vi "GenCtrlCsv.vi"(6 "Loop Time (s)":dbl, 7 "Gen Control":T1, 8 "error in (no error)":errorcluster, 9 "ROSCO Params in":T6, 10 "IO Signals In":T5, 11 "ArrayPairs In":T3={"iStatus"={"Index"=0, "Value"=0.0}, "TIME"={"Index"=1, "Value"=0.0}, "DT"={"Index"=2, "Value"=0.0}, "Blade1PitchPos_rad"={"Index"=3, "Value"=0.0}, "VS_MECHGENPWR"={"Index"=13, "Value"=0.0}, "VS_GENPWR"={"Index"=14, "Value"=0.0}, "GEN_SPEED"={"Index"=19, "Value"=0.0}, "ROTOR_SPEED"={"Index"=20, "Value"=0.0}, "GENTQMEAS"={"Index"=22, "Value"=0.0}, "Y_M"={"Index"=23, "Value"=0.0}, "HORWINDV"={"Index"=26, "Value"=0.0}, "ROOTMOOP1"={"Index"=29, "Value"=0.0}, "ROOTMOOP2"={"Index"=30, "Value"=0.0}, "Blade2PitchPos_rad"={"Index"=32, "Value"=0.0}, "Blade3PitchPos_rad"={"Index"=33, "Value"=0.0}, "ROOTMOOP3"={"Index"=31, "Value"=0.0}, "AVCMSG_SIZE"={"Index"=48, "Value"=0.0}, "INFILE_SIZE "={"Index"=49, "Value"=0.0}, "OUTFILE_SIZE "={"Index"=50, "Value"=0.0}, "FA_ACC"={"Index"=52, "Value"=0.0}, "NUM_BLADES"={"Index"=60, "Value"=0.0}, "BladePitchSetpoint_rad"={"Index"=44, "Value"=0.0}, "TorqueSetpoint_Nm"={"Index"=46, "Value"=0.0}, "OUT_AEROTQ"={"Index"=89, "Value"=0.0}, "Out.RotSpeed "={"Index"=92, "Value"=0.0}, "Out.DEBUG"={"Index"=93, "Value"=0.0}}) -> (0 "error out":errorcluster, 1 "ROSCO Params Out":T6, 2 "IO Signals Out":T5, 3 "ArrayPairs Out":T3={"iStatus"={"Index"=0, "Value"=0.0}, "TIME"={"Index"=1, "Value"=0.0}, "DT"={"Index"=2, "Value"=0.0}, "Blade1PitchPos_rad"={"Index"=3, "Value"=0.0}, "VS_MECHGENPWR"={"Index"=13, "Value"=0.0}, "VS_GENPWR"={"Index"=14, "Value"=0.0}, "GEN_SPEED"={"Index"=19, "Value"=0.0}, "ROTOR_SPEED"={"Index"=20, "Value"=0.0}, "GENTQMEAS"={"Index"=22, "Value"=0.0}, "Y_M"={"Index"=23, "Value"=0.0}, "HORWINDV"={"Index"=26, "Value"=0.0}, "ROOTMOOP1"={"Index"=29, "Value"=0.0}, "ROOTMOOP2"={"Index"=30, "Value"=0.0}, "Blade2PitchPos_rad"={"Index"=32, "Value"=0.0}, "Blade3PitchPos_rad"={"Index"=33, "Value"=0.0}, "ROOTMOOP3"={"Index"=31, "Value"=0.0}, "AVCMSG_SIZE"={"Index"=48, "Value"=0.0}, "INFILE_SIZE "={"Index"=49, "Value"=0.0}, "OUTFILE_SIZE "={"Index"=50, "Value"=0.0}, "FA_ACC"={"Index"=52, "Value"=0.0}, "NUM_BLADES"={"Index"=60, "Value"=0.0}, "BladePitchSetpoint_rad"={"Index"=44, "Value"=0.0}, "TorqueSetpoint_Nm"={"Index"=46, "Value"=0.0}, "OUT_AEROTQ"={"Index"=89, "Value"=0.0}, "Out.RotSpeed "={"Index"=92, "Value"=0.0}, "Out.DEBUG"={"Index"=93, "Value"=0.0}}, 4 "Velocity setpoint (rad/s)":dbl, 5 "Torque setpoint (Nm)":dbl)   [LabVIEW 2018]
uses:
  Clusters/RoscoParams.ctl
  Clusters/IOSignals.ctl
  Clusters/ArrayPairs.ctl
  Clusters/SwapArrayCluster.ctl
  Clusters/GenCtrl.ctl
  Clusters/GenMode.ctl
  Clusters/GenCtrlMode.ctl
  <vilib>/addons/control/pid/pid.llb/PID Output Rate Limiter (DBL).vi
  <vilib>/addons/control/pid/NI_PID_pid.lvlib
panel:
  out "Current ramp time (s)":dbl
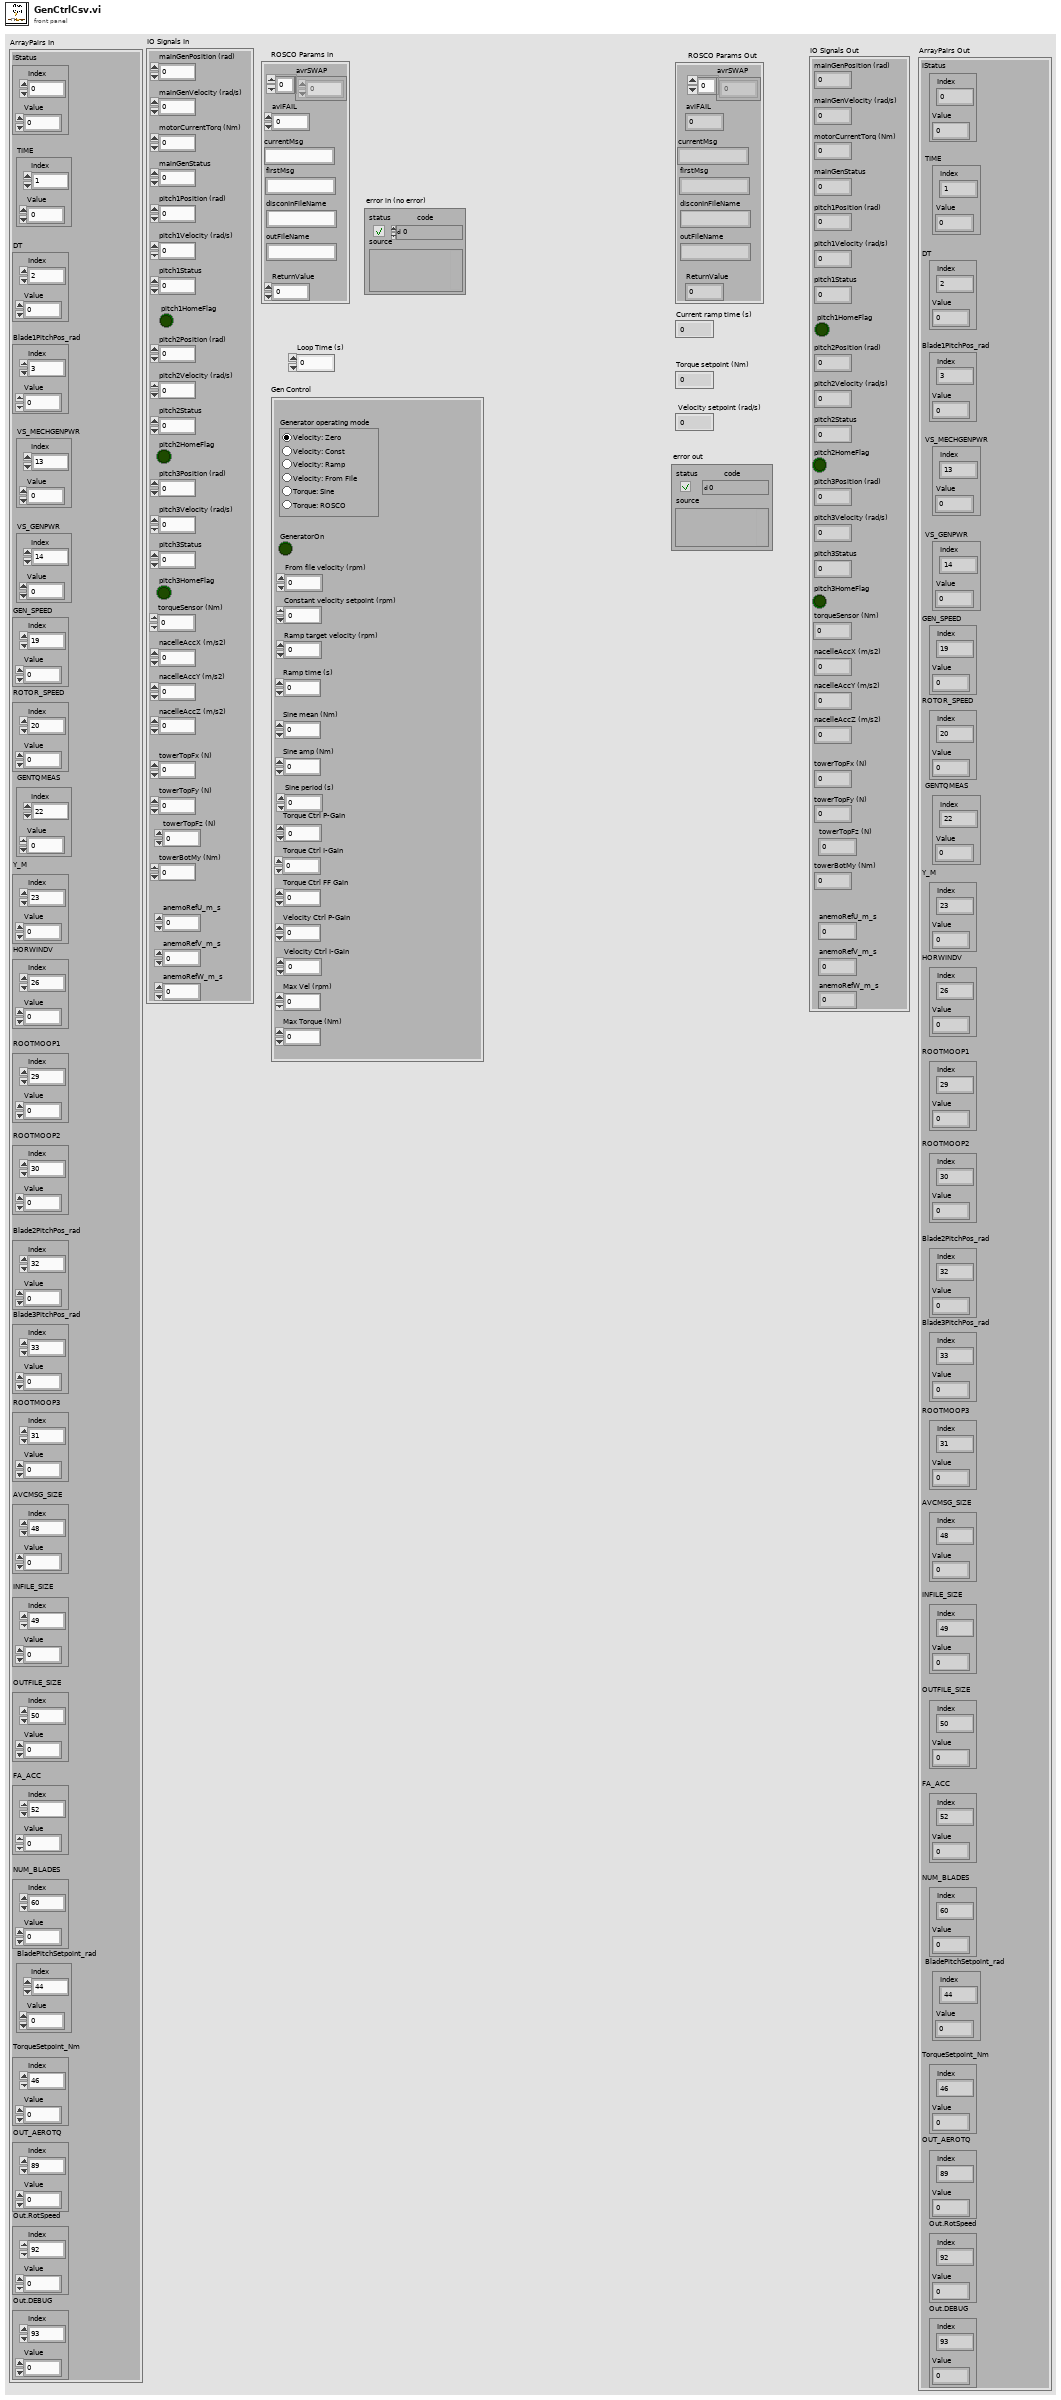
[diagram p1: front panel]
types:
  T1 = typedef "GenCtrl.ctl" = cluster{"Constant velocity setpoint (rpm)":dbl, "Ramp target velocity (rpm)":dbl, "Ramp time (s)":dbl, "Sine mean (Nm)":dbl, "Sine amp (Nm)":dbl, "Sine period (s)":dbl, "Torque Ctrl I-Gain":dbl, "Velocity Ctrl P-Gain":dbl, "Velocity Ctrl I-Gain":dbl, "Max Torque (Nm)":dbl, "GeneratorOn":bool, "Torque Ctrl P-Gain":dbl, "From file velocity (rpm)":dbl, "Generator operating mode":T2, "Max Vel (rpm)":dbl, "Torque Ctrl FF Gain":dbl}
  T2 = typedef "GenMode.ctl" = enum32{"Velocity: Zero", "Velocity: Const.", "Velocity: Ramp", "Velocity: From File", "Torque: Sine", "Torque: ROSCO"}
  T3 = typedef "ArrayPairs.ctl" = cluster{"iStatus":T4, "TIME":T4, "DT":T4, "Blade1PitchPos_rad":T4, "VS_MECHGENPWR":T4, "VS_GENPWR":T4, "GEN_SPEED":T4, "ROTOR_SPEED":T4, "GENTQMEAS":T4, "Y_M":T4, "HORWINDV":T4, "ROOTMOOP1":T4, "ROOTMOOP2":T4, "Blade2PitchPos_rad":T4, "Blade3PitchPos_rad":T4, "ROOTMOOP3":T4, "AVCMSG_SIZE":T4, "INFILE_SIZE ":T4, "OUTFILE_SIZE ":T4, "FA_ACC":T4, "NUM_BLADES":T4, "BladePitchSetpoint_rad":T4, "TorqueSetpoint_Nm":T4, "OUT_AEROTQ":T4, "Out.RotSpeed ":T4, "Out.DEBUG":T4}
  T4 = typedef "SwapArrayCluster.ctl" = cluster{"Index":i32, "Value":dbl}
  T5 = typedef "IOSignals.ctl" = cluster{"mainGenPosition (rad)":dbl, "motorCurrentTorq (Nm)":dbl, "mainGenVelocity (rad/s)":dbl, "mainGenStatus":u16, "pitch1Position (rad)":dbl, "pitch1Velocity (rad/s)":dbl, "pitch1Status":u16, "pitch2Position (rad)":dbl, "pitch2Velocity (rad/s)":dbl, "pitch2Status":u16, "pitch3Position (rad)":dbl, "pitch3Velocity (rad/s)":dbl, "pitch3Status":u16, "torqueSensor (Nm)":dbl, "nacelleAccX (m/s2)":dbl, "nacelleAccY (m/s2)":dbl, "nacelleAccZ (m/s2)":dbl, "pitch1HomeFlag":bool, "pitch2HomeFlag":bool, "pitch3HomeFlag":bool, "towerTopFx (N)":dbl, "towerTopFy (N)":dbl, "towerTopFz (N)":dbl, "towerBotMy (Nm)":dbl, "anemoRefU_m_s":dbl, "anemoRefV_m_s":dbl, "anemoRefW_m_s":dbl}
  T6 = typedef "RoscoParams.ctl" = cluster{"avrSWAP":dbl[], "aviFAIL":i32, "currentMsg":string, "ReturnValue":i32, "disconInFileName":string, "outFileName":string, "firstMsg":string}
  T7 = typedef "GenCtrlMode.ctl" = enum16{"Torque Control", "Velocity Control"}
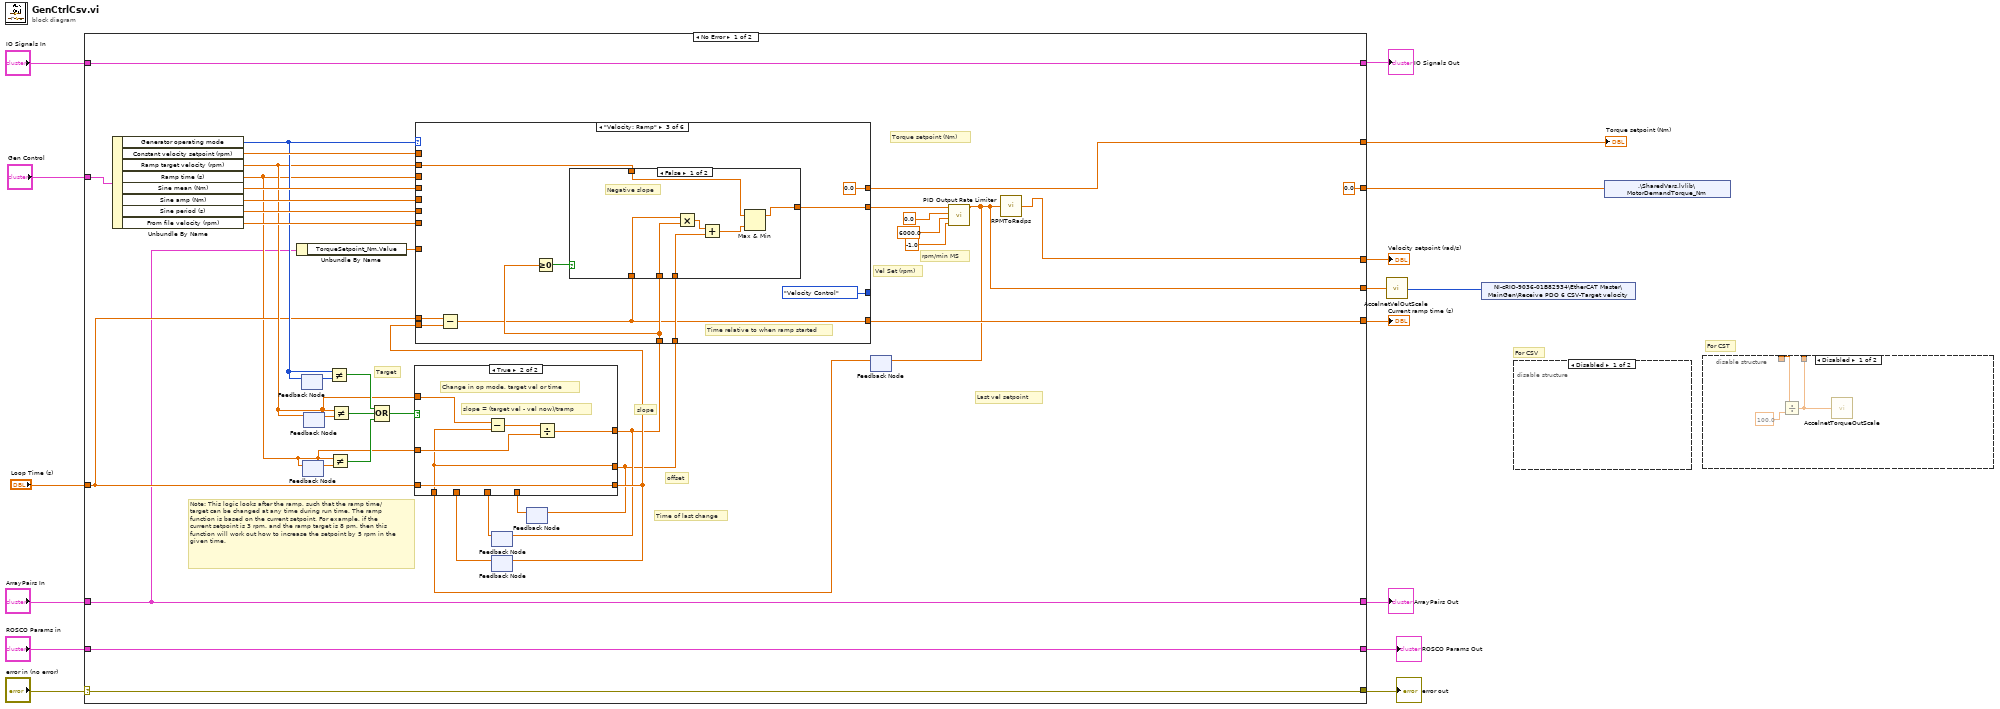
[diagram p0: block diagram]
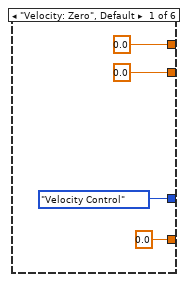
[diagram p5: hidden frame]
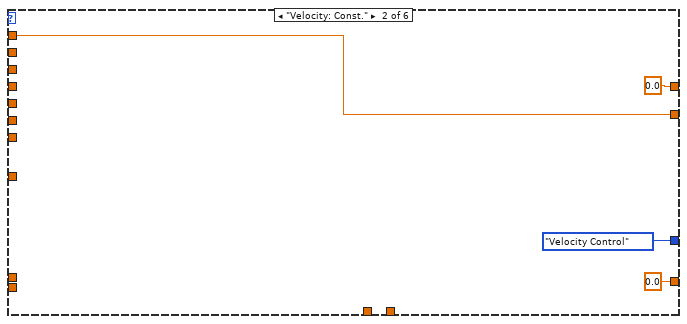
[diagram p6: hidden frame]
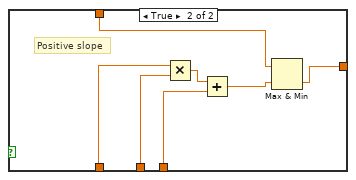
[diagram p7: hidden frame]
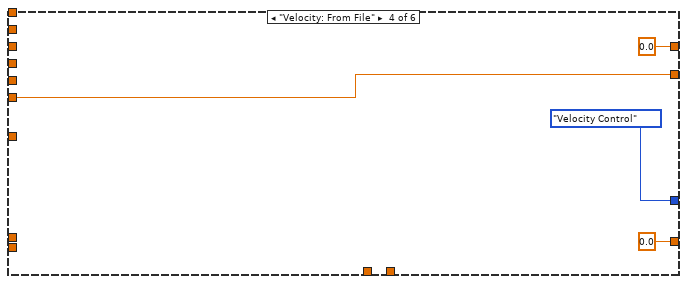
[diagram p8: hidden frame]
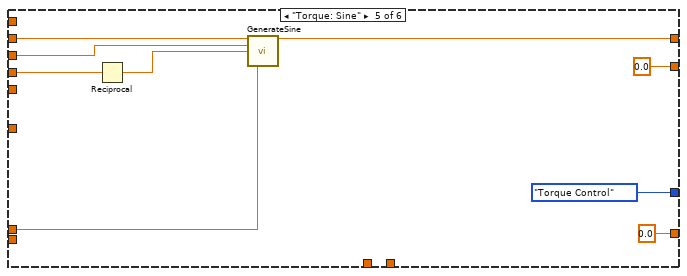
[diagram p9: hidden frame]
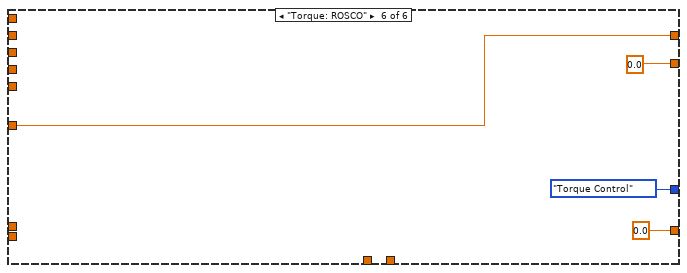
[diagram p10: hidden frame]
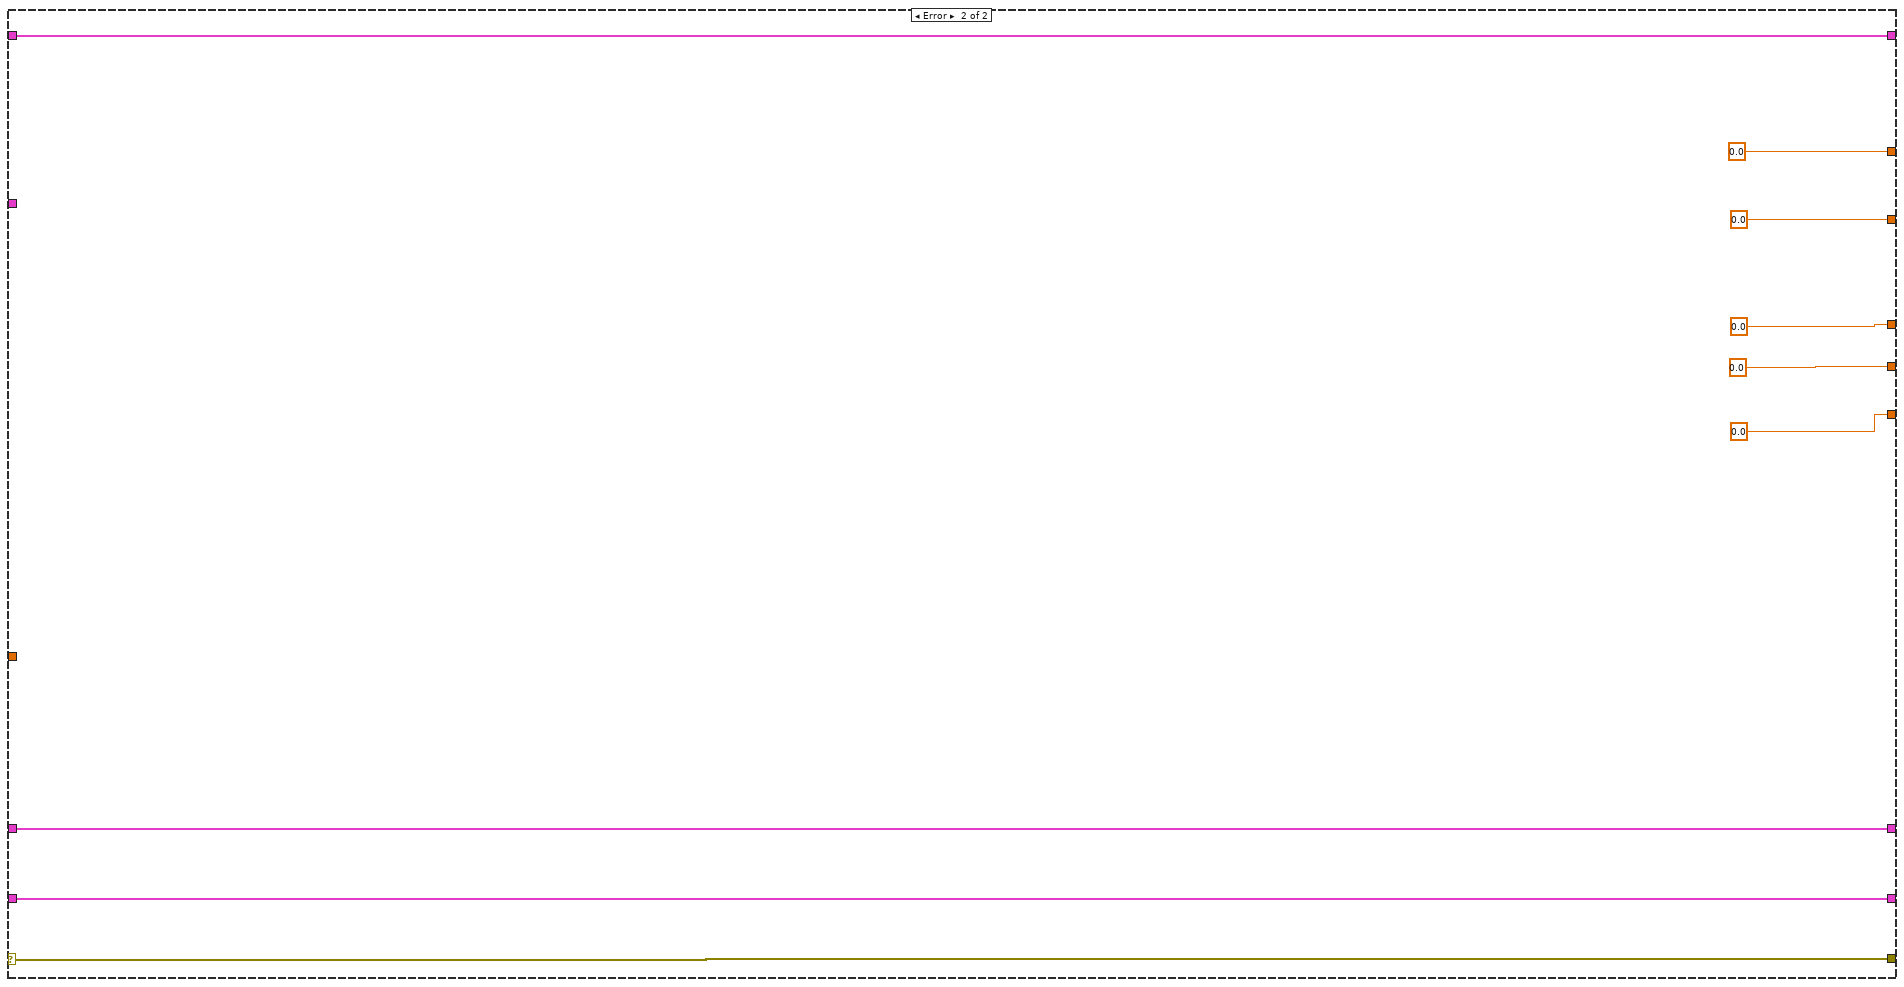
[diagram p11: hidden frame]
diagram:
  # "For CST"
  # "For CSV"
  n1 = case shown="No Error" "error in (no error)" {
    selector: "error in (no error)" -> [w53 w121]
    tunnel: [w53 w121] -> w15
    tunnel: [w54 w120] -> w13
    tunnel: "ROSCO Params in" -> [w54 w120]
    tunnel: [w24 w119] -> w11
    tunnel: "ArrayPairs In" -> [w24 w119]
    tunnel: [w50 w118] -> w9
    tunnel: "IO Signals In" -> [w50 w118]
    tunnel: "Loop Time (s)" -> [w33 _]
    tunnel: "Gen Control" -> [w46 _]
    tunnel: [w51 0.0 ("Loop Time (s)")] -> w5
    tunnel: [0.0 0.0] -> w1
    tunnel: [w27 0.0 ("Constant velocity setpoint (rpm)")] -> w6
    tunnel: [w45 0.0 ("Constant velocity setpoint (rpm)")] -> w4
    tunnel: [w18 0.0 ("output")] -> w3
    frame No Error {
      # "rpm/min MS"
      # "Note: This logic looks after the ramp, such that the ramp time/target can be changed at any time during run time. The ramp function is based on the current setpoint. For example, if the current setpoint is 3 rpm. and the ramp target is 8 pm, then this function will work out how to increase the setpoint by 5 rpm in the given time."
      # "offset"
      # "slope"
      # "Last vel setpoint"
      # "Time of last change"
      # "Target"
      # "Vel Set (rpm)"
      # "Torque setpoint (Nm)"
      n2 = Unbundle By Name(w46) -> ("Generator operating mode"=w43:T2, "Constant velocity setpoint (rpm)"=w52:dbl, "Ramp target velocity (rpm)"=w35:dbl, "Ramp time (s)"=w31:dbl, "Sine mean (Nm)"=w49:dbl, "Sine amp (Nm)"=w48:dbl, "Sine period (s)"=w47:dbl, "From file velocity (rpm)"=w44:dbl)
      n3 = Unbundle By Name(w24) -> ("TorqueSetpoint_Nm.Value"=w23:dbl)
      n4 = feedback-in #1(w43) -> ()
      n5 = feedback #1() -> (w42:T2)  [unwired: 1 in]
      n6 = feedback #2() -> (w40:dbl)  [unwired: 1 in]
      n7 = feedback-in #2(w31) -> ()
      n8 = feedback #3() -> (w41:dbl)  [unwired: 1 in]
      n9 = feedback-in #3(w35) -> ()
      n10 = Not Equal?(x=w43, y=w42) -> (x != y?=w37:bool)
      n11 = Not Equal?(x=w31, y=w40) -> (x != y?=w39:bool)
      n12 = Not Equal?(x=w35, y=w41) -> (x != y?=w38:bool)
      n13 = Compound Arithmetic op=OR(w37, w38, w39) -> (w36:bool)
      n14 = feedback #4() -> (w29:dbl)  [unwired: 1 in]
      n15 = feedback #5() -> (w34:dbl)  [unwired: 1 in]
      n16 = feedback #6() -> (w25:dbl)  [unwired: 1 in]
      n17 = feedback #7() -> (w28:dbl)  [unwired: 1 in]
      n18 = case shown="True" w36 {
        tunnel: w28 -> [_ w58]
        tunnel: w35 -> [_ w62]
        tunnel: w33 -> [_ w63]
        tunnel: [w57 w63] -> w32
        tunnel: w34 -> [w57 _]
        tunnel: w31 -> [_ w60]
        tunnel: [w56 w59] -> w30
        tunnel: w29 -> [w56 _]
        tunnel: [w55 w58] -> w26
        tunnel: w25 -> [w55 _]
        frame False {
        }
        frame True {
          # "slope = (target vel - vel now)/tramp"
          # "Change in op mode, target vel or time"
          n19 = Subtract(x=w62, y=w58) -> (x-y=w61:dbl)
          n20 = Divide(x=w61, y=w60) -> (x/y=w59:dbl)
        }
      }
      n21 = case shown="\"Velocity: Ramp\"" w43 {
        tunnel: w52 -> [_ w68 _ _ _ _]
        tunnel: w35 -> [_ _ w73 _ _ _]
        tunnel: w31 -> [_ _ _ _ _ _]
        tunnel: [0.0 ("Constant velocity setpoint (rpm)") 0.0 ("Constant velocity setpoint (rpm)") w74 0.0 ("Constant velocity setpoint (rpm)") 0.0 ("Constant velocity setpoint (rpm)") 0.0 ("Constant velocity setpoint (rpm)")] -> w51
        tunnel: w49 -> [_ _ _ _ w107 _]
        tunnel: [0.0 ("Constant velocity setpoint (rpm)") 0.0 ("Constant velocity setpoint (rpm)") 0.0 ("Constant torque setpoint (Nm)") 0.0 ("Constant torque setpoint (Nm)") w100 w109] -> w45
        tunnel: w48 -> [_ _ _ _ w106 _]
        tunnel: w47 -> [_ _ _ _ w105 _]
        tunnel: [0.0 ("Constant velocity setpoint (rpm)") w68 w72 w96 0.0 ("Constant velocity setpoint (rpm)") 0.0 ("Constant velocity setpoint (rpm)")] -> w19
        tunnel: [GenCtrlMode."Velocity Control" GenCtrlMode."Velocity Control" GenCtrlMode."Velocity Control" GenCtrlMode."Velocity Control" GenCtrlMode."Torque Control" GenCtrlMode."Torque Control"] -> _
        tunnel: w44 -> [_ _ _ w96 _ _]
        tunnel: w33 -> [_ _ w79 _ w101 _]
        tunnel: w32 -> [_ _ w78 _ _ _]
        tunnel: w30 -> [_ _ w75 _ _ _]
        tunnel: w26 -> [_ _ w76 _ _ _]
        tunnel: w23 -> [_ _ _ _ _ w109]
        frame "Velocity: Zero", Default {
        }
        frame "Velocity: Const." {
        }
        frame "Velocity: Ramp" {
          # "Time relative to when ramp started"
          n22 = Subtract(x=w79, y=w78) -> (x-y=w74:dbl)
          n23 = Greater Or Equal To 0?(x=w75) -> (x >= 0?=w77:bool)
          n24 = case shown="False" w77 {
            tunnel: w76 -> [w85 w92]
            tunnel: w75 -> [w87 w93]
            tunnel: w74 -> [w88 w94]
            tunnel: w73 -> [w83 w90]
            tunnel: [w82 w89] -> w72
            frame False {
              # "Negative slope"
              n25 = Multiply(x=w88, y=w87) -> (x*y=w86:dbl)
              n26 = Add(x=w86, y=w85) -> (x+y=w84:dbl)
              n27 = Max & Min(x=w83, y=w84) -> (max(x,y)=w82:dbl)  [unwired: 1 out]
            }
            frame True {
              # "Positive slope"
              n28 = Multiply(x=w94, y=w93) -> (x*y=w95:dbl)
              n29 = Add(x=w95, y=w92) -> (x+y=w91:dbl)
              n30 = Max & Min(x=w90, y=w91) -> (min(x,y)=w89:dbl)  [unwired: 1 out]
            }
          }
        }
        frame "Velocity: From File" {
        }
        frame "Torque: Sine" {
          n31 = Reciprocal(x=w105) -> (1/x=w104:dbl)
          n32 = call "GenerateSine.vi"("Mean"=w107, "Amplitude"=w106, "frequency (f)"=w104, "time (s)"=w101) -> ("sine out"=w100:dbl)  [unwired: 11 in]
        }
        frame "Torque: ROSCO" {
        }
      }
      n33 = feedback-in #4(w30) -> ()
      n34 = feedback-in #5(w32) -> ()
      n35 = feedback-in #6(w26) -> ()
      n36 = call-poly <vilib>:"PID Output Rate Limiter.vi"("dt (s)"=-1.0, "output rate (EGU/min)"=6000.0, "initial output"=0.0, "input (controller output)"=w19) -> ("output"=w18:dbl)  [unwired: 4 in, 1 out]
      n37 = feedback-in #7(w18) -> ()
      n38 = call "RPMToRadps.vi"("rpm"=w18) -> ("rad/s"=w27:dbl)
    }
    frame Error {
    }
  }
  "error out" <- w15
  "ROSCO Params Out" <- w13
  "IO Signals Out" <- w9
  "ArrayPairs Out" <- w11
  "Current ramp time (s)" <- w5
  "Torque setpoint (Nm)" <- w4
  "Velocity setpoint (rad/s)" <- w6
  n39 = call "AccelnetVelOutScale.vi"("Shaft vel (rpm)"=w3) -> ("Acelnet eCAT vel"=w2:i32)
  n40 = shared-variable "NI-cRIO-9036-01B82934\\EtherCAT Master\\MainGen\\Receive PDO 6 CSV-Target velocity"(w2) -> ()  [unwired: 1 in, 1 out]
  n41 = disable-structure shown="Disabled" {
    frame Disabled {
    }
    frame Enabled {
    }
  }
  n42 = shared-variable ".\\SharedVars.lvlib\\MotorDemandTorque_Nm"(w1) -> ()  [unwired: 1 in, 1 out]
  n43 = disable-structure shown="Disabled" {
    disable-tunnel: _ -> [w123 _]
    disable-tunnel: [w122 _] -> _
    frame Disabled {
      n44 = Divide(x=w123, y=100.0) -> (x/y=w122:dbl)
      n45 = call "AccelnetTorqueOutScale.vi"("Demand torque (Nm)"=w122) -> ()  [unwired: 1 out]
    }
    frame Enabled {
    }
  }
